vi "Listage_NumeroStockes_OK.vi"(0 "Fichier ou dossier Reseau":path=path "C:/TEST/réseaux", 1 "nbr de sous dossier":i32=4, 5 "Dossier Local":path=path "C:/TEST/Local", 11 "error in":errorcluster caption="entrée d'erreur (pas d'erreur)") -> (4 "Liste pièces stockées OK":string[](array[string]), 15 "error out":errorcluster)   [LabVIEW 2020]
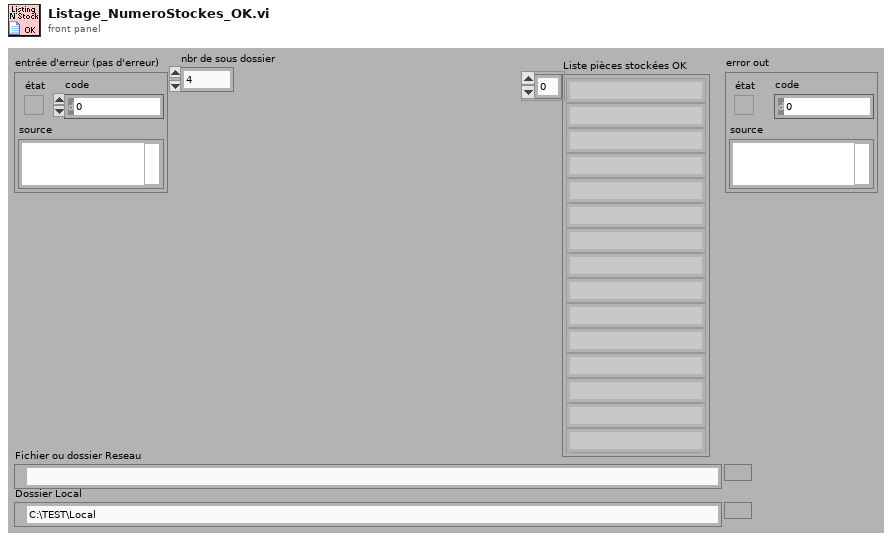
[diagram p1: front panel]
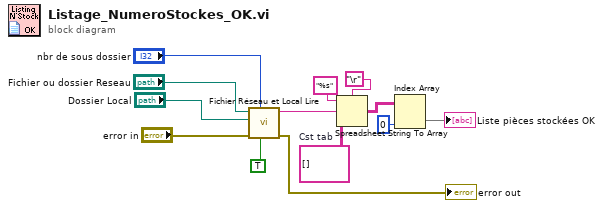
[diagram p0: block diagram]
diagram:
  w10 = string[][] []  # Cst tab
  n1 = call "Fichier Réseau et Local Lire .vi"("reseau prioritaire ?"=TRUE, "nbr de sous dossier"="nbr de sous dossier", "error in"="error in", "Dossier Local"="Dossier Local", "Fichier ou dossier Reseau"="Fichier ou dossier Reseau") -> ("error out"=→"error out":errorcluster, "Texte"=w12:string)  [unwired: 2 in, 2 out]
  n2 = Spreadsheet String To Array(delimiter (Tab)="\r", format string="%s", spreadsheet string=w12, array type (2D Dbl)=w10) -> (array=w5:string[][])
  n3 = Index Array(array=w5, index (col)=0 ("indice désactivé (col)")) -> (element=→"Liste pièces stockées OK":string[])  [unwired: 1 in]
